vi "LabviewEnvsInstalled.vi"   [LabVIEW 2020]
uses:
  <vilib>/Wiresmith Technology/G CLI/Argument Parser/Option Class/Option Configuration.ctl
  <vilib>/Wiresmith Technology/G CLI/Argument Parser/Option Class/Argument Type.ctl
  <vilib>/Utility/error.llb/DialogType.ctl
  094f6021-4ef8-4573-82ce-a7b4949f6c5c.vi
  67a138f0-9744-4b2d-9c21-223ad79f4533.vi
  6795289f-0a04-455c-a499-a5e59a361415.vi
  <vilib>/JDP Science/JSONtext/Variant to JSON Text.vi
  <vilib>/JDP Science/JSONtext/LVClass Serializer/JSONtext LVClass Serializer.lvclass
  <vilib>/Wiresmith Technology/G CLI/CLI Class/CLI.lvclass
  <vilib>/Wiresmith Technology/G CLI/Argument Parser/Option Set Class/Option Set.lvclass
  <vilib>/Wiresmith Technology/G CLI/Argument Parser/Option Class/Option.lvclass
  <vilib>/JDP Science/JSONtext/JSONtext.lvlib
types:
  T1 = enum32{"Invalid", "Standard", "Closed", "Hidden", "Minimized", "Maximized"}
  T2 = typedef "Option Parser.lvlib/Option.lvclass/Option Configuration.ctl" = cluster{"Option Type":T3, "Option Labels":string[], "Key":string, "Description":string, "Required":bool, "Default Value":string}
  T3 = typedef "Option Parser.lvlib/Option.lvclass/Argument Type.ctl" = enum16{"flag", "value"}
  T4 = typedef "LabViewApplication--cluster.ctl" = cluster{"Bitness":enum8{"Unknown", "x86", "x64"}, "Version":string, "LabVIEW.exe":path, "VersionString":string}
  T5 = typedef "DialogType.ctl" = u16
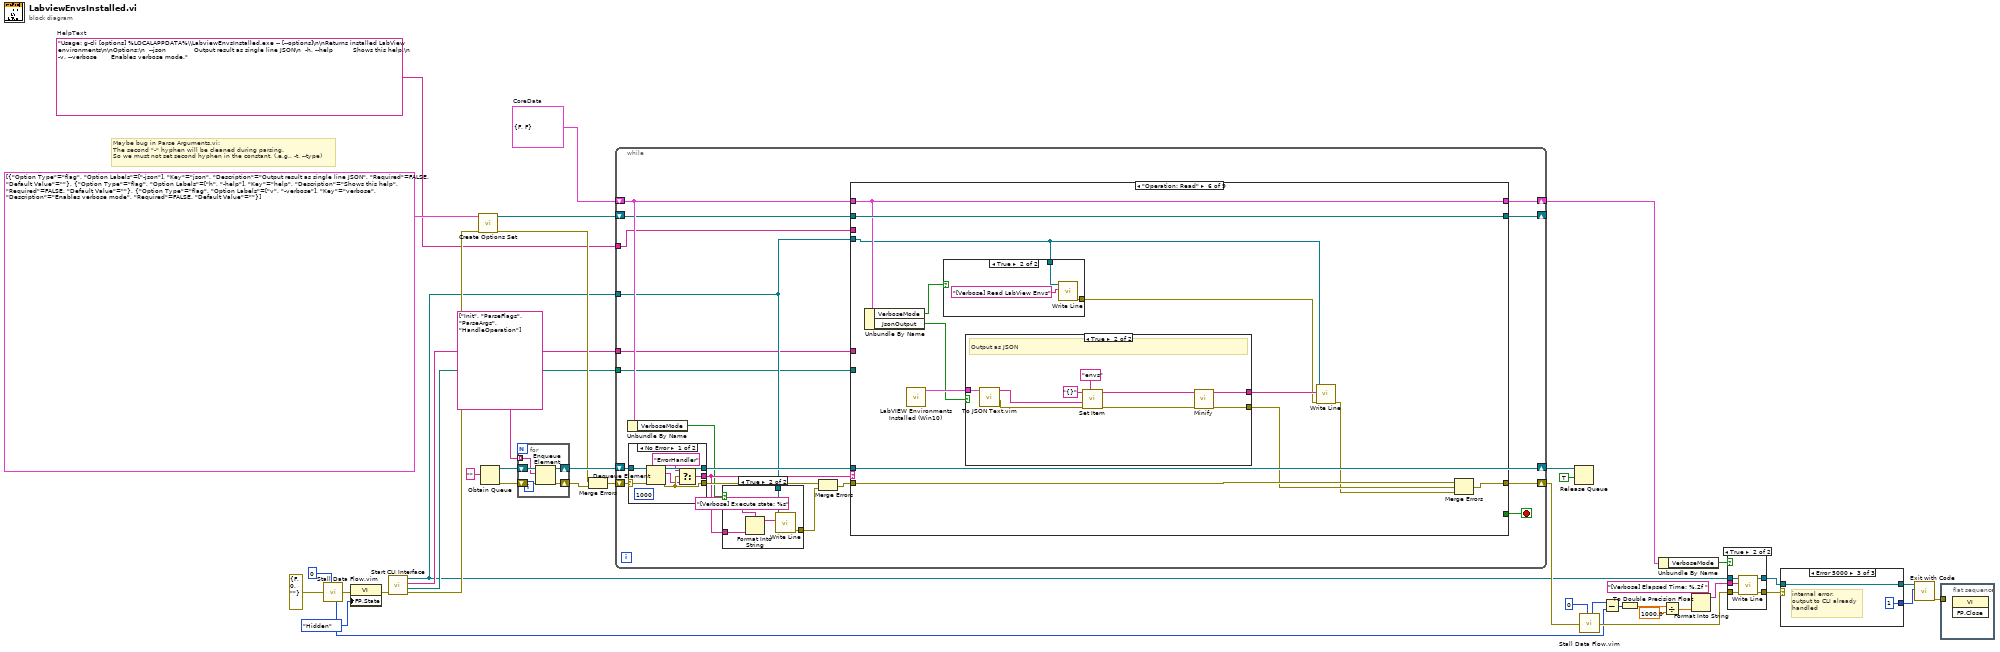
[diagram p0: block diagram]
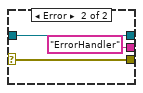
[diagram p4: hidden frame]
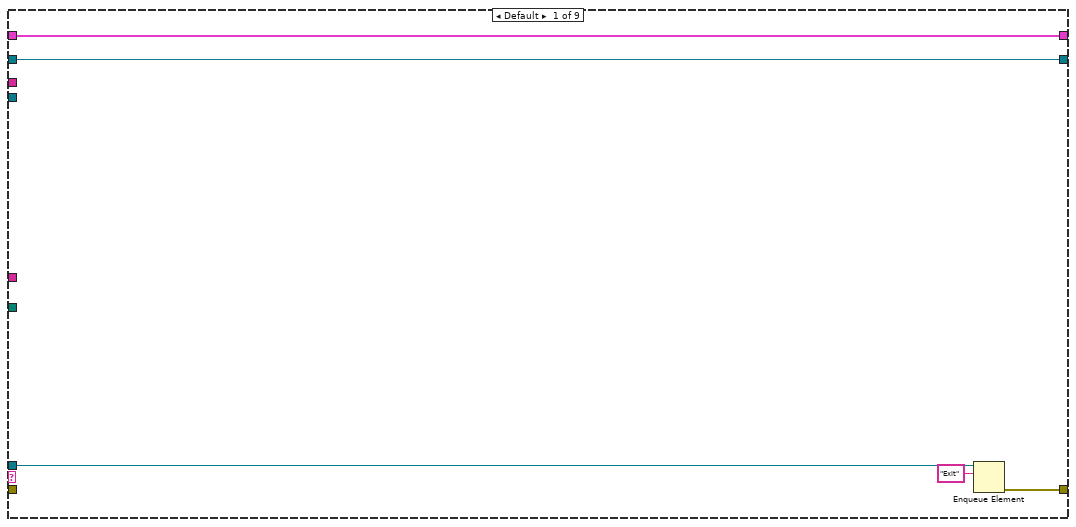
[diagram p5: hidden frame]
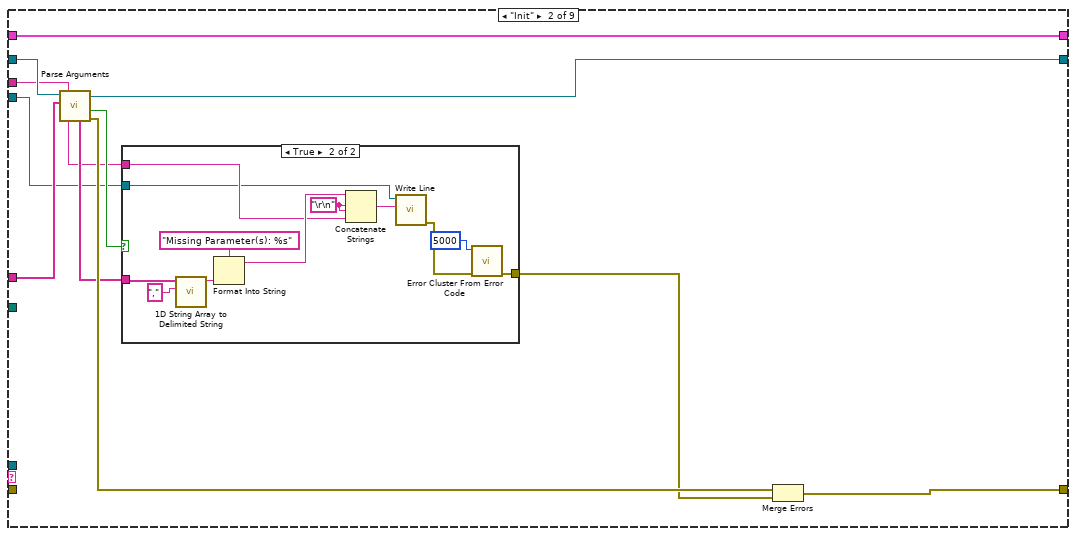
[diagram p6: hidden frame]
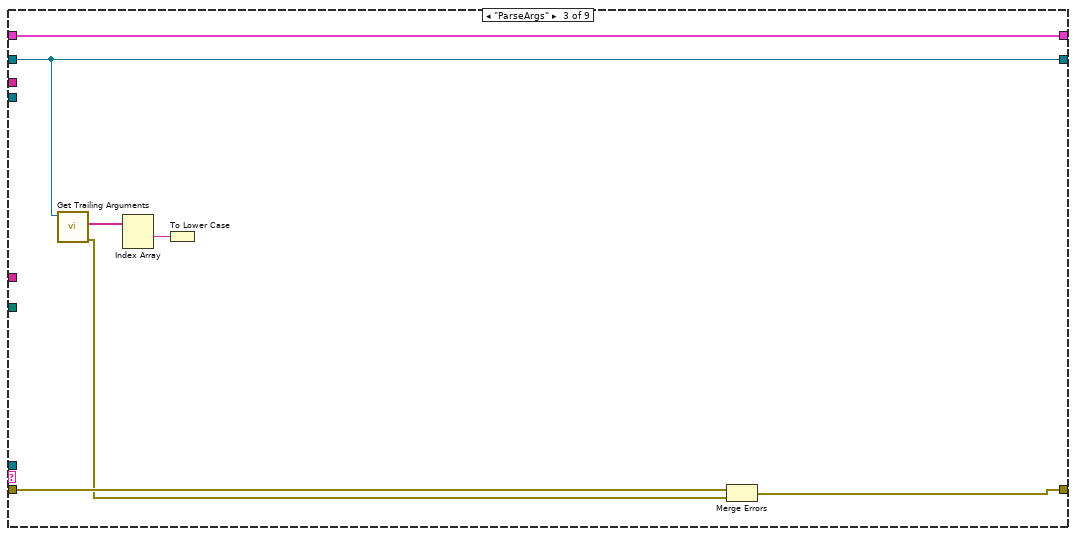
[diagram p8: hidden frame]
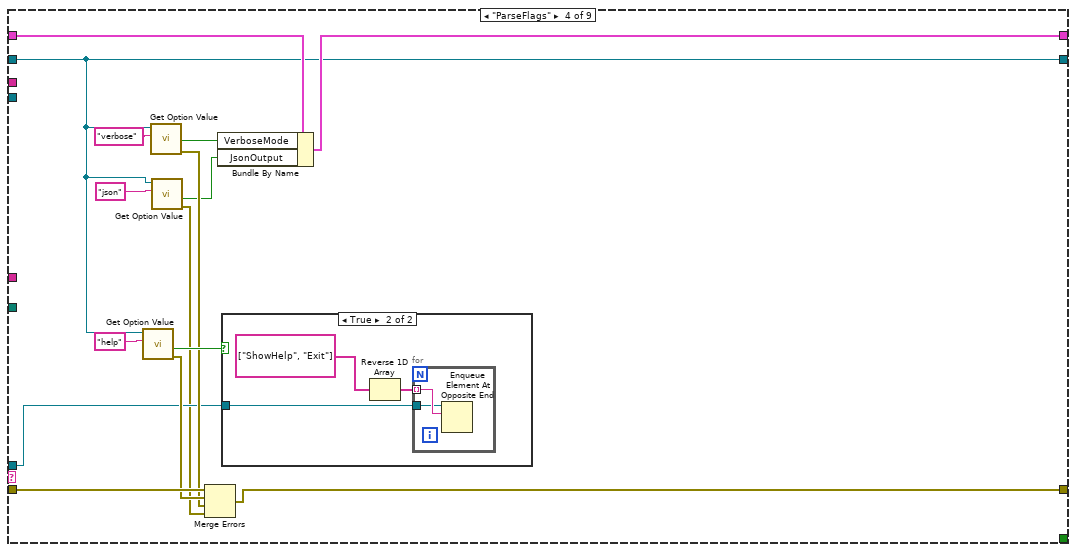
[diagram p9: hidden frame]
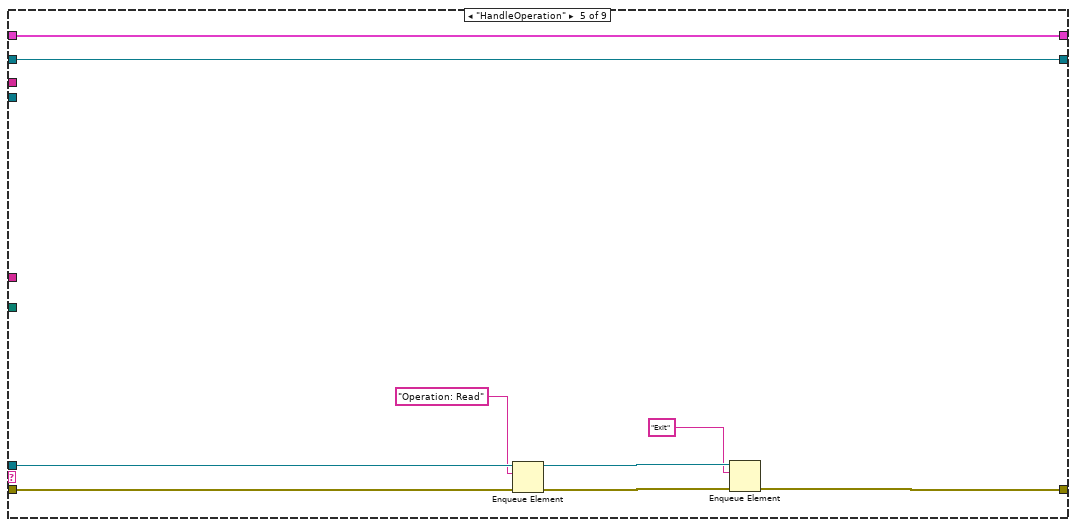
[diagram p11: hidden frame]
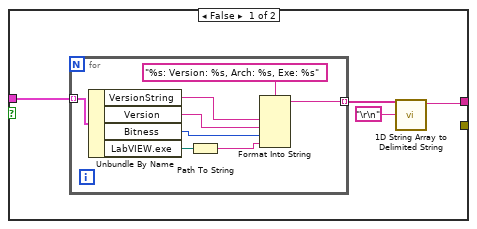
[diagram p12: hidden frame]
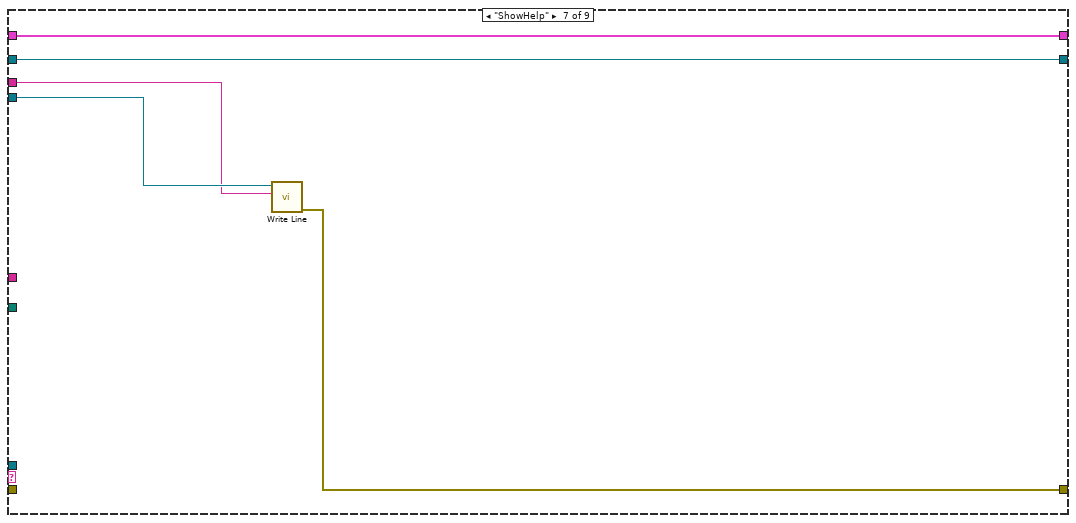
[diagram p14: hidden frame]
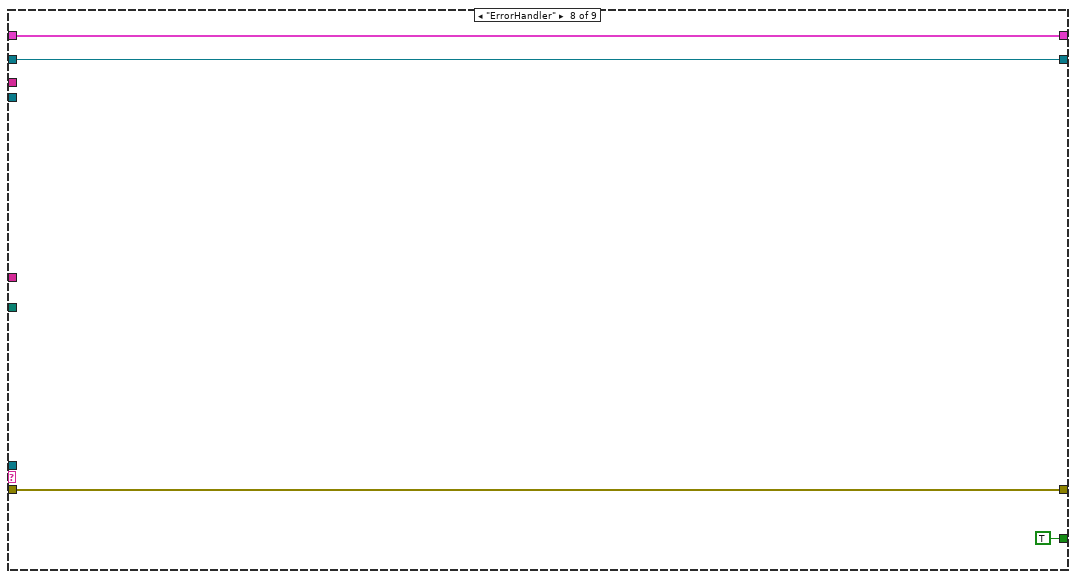
[diagram p15: hidden frame]
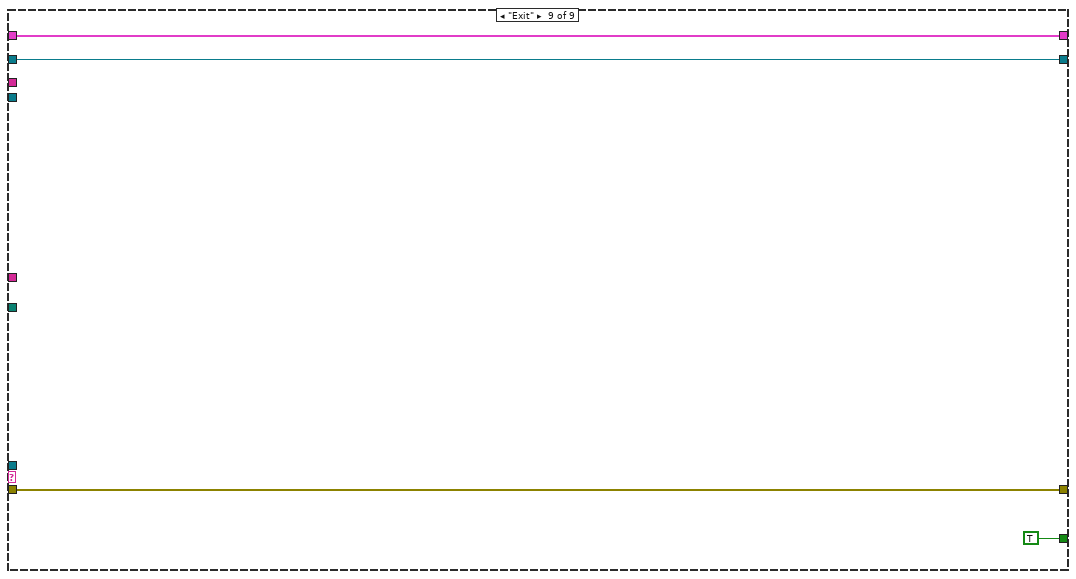
[diagram p16: hidden frame]
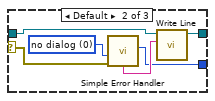
[diagram p18: hidden frame]
diagram:
  w1 = "Usage: g-cli [options] %LOCALAPPDATA%\\LabviewEnvsInstalled.exe -- [--options]\n\nReturns installed LabView environments\n\nOptions:\n  --json              Output result as single line JSON\n  -h, --help          Shows this help.\n  -v, --verbose       Enables verbose mode."  # HelpText
  w14 = cluster{"VerboseMode":bool, "JsonOutput":bool} {"VerboseMode"=FALSE, "JsonOutput"=FALSE}  # CoreData
  # "Maybe bug in Parse Arguments.vi: \nThe second \"-\" hyphen will be cleaned during parsing.\nSo we must not set second hyphen in the constant. (.e.g., -t, --type)"
  n1 = call "Stall Data Flow.vim"("value in"=errorcluster {"status"=FALSE, "code"=0, "source"=""} ("error in (no error)"), "milliseconds to wait"=u32 0) -> ("millisecond timer value"=w30:u32, "value out"=w37:errorcluster)
  n2 = property class="VI"(error in=w37, "FP.State"=T1."Hidden" ("Front Panel Window:State")) -> (error out=w36:errorcluster)  [unwired: 1 in, 1 out]
  n3 = call <vilib>:"Start CLI Interface.vi"("error in (no error)"=w36) -> ("error out"=w41:errorcluster, "Working Directory"=w7:path, "Custom Parameters"=w8:string[], "CLI out"=w5:refnum<class "CLI.lvclass">)  [unwired: 7 in]
  n4 = call <vilib>:"Create Options Set.vi"("error in (no error)"=w41, "Options"=T2[] [{"Option Type"=enum."flag", "Option Labels"=["-json"], "Key"="json", "Description"="Output result as single line JSON", "Required"=FALSE, "Default Value"=""}, {"Option Type"=enum."flag", "Option Labels"=["h", "-help"], "Key"="help", "Description"="Shows this help", "Required"=FALSE, "Default Value"=""}, {"Option Type"=enum."flag", "Option Labels"=["v", "-verbose"], "Key"="verbose", "Description"="Enables verbose mode", "Required"=FALSE, "Default Value"=""}]) -> ("error out"=w10:errorcluster, "Option Set out"=w12:refnum<class "Option Set.lvclass">)  [unwired: 8 in]
  n5 = Obtain Queue(element data type="") -> (queue out=w19:refnum<queue>, error out=w16:errorcluster)  [unwired: 4 in, 1 out]
  n6 = for {
    shift-right: [w45] -> w17
    shift-left: w19 -> [w46]
    shift-right: [w43] -> w11
    shift-left: w16 -> [w44]
    tunnel: string[] ["Init", "ParseFlags", "ParseArgs", "HandleOperation"] -> [w42] mode=indexing
    n7 = Enqueue Element(queue=w46, element=w42, error in (no error)=w44) -> (queue out=w45:refnum<queue>, error out=w43:errorcluster)  [unwired: 1 in, 1 out]
  }
  n8 = Merge Errors(w10, w11) -> (w9:errorcluster)
  n9 = while {
    shift-right: [w61] -> w4
    shift-left: w14 -> [w56]
    shift-right: [w59] -> w6
    shift-left: w9 -> [w63]
    shift-right: [w58] -> w15
    shift-left: w17 -> [w64]
    tunnel: w5 -> [w54]
    tunnel: w8 -> [w49]
    tunnel: w7 -> [w50]
    tunnel: w1 -> [w48]
    shift-right: [w47] -> _
    shift-left: w12 -> [w53]
    stop <- w60 stop-if-true
    n10 = Unbundle By Name(w56) -> ("VerboseMode"=w55:bool)
    n11 = case shown="No Error" w63 {
      selector: w63 -> [w75 w79]
      tunnel: w64 -> [w76 w78]
      tunnel: [w71 "ErrorHandler"] -> w57
      tunnel: [w73 w79] -> w62
      tunnel: [w74 w78] -> w58
      frame No Error {
        (unwired) 1000 ("timeout in ms (-1)")
        n12 = Dequeue Element(queue=w76, error in (no error)=w75) -> (queue out=w74:refnum<queue>, element=w72:string, error out=w73:errorcluster)  [unwired: 1 in, 1 out]
        n13 = Select(t="ErrorHandler", s=w73, f=w72) -> (s? t:f=w71:string)
      }
      frame Error {
      }
    }
    n14 = case shown="True" w55 {
      tunnel: w57 -> [_ w69]
      tunnel: w54 -> [_ w66]
      tunnel: [_ w65] -> w51
      frame False {
      }
      frame True {
        n15 = Format Into String(format string="[Verbose] Execute state: %s", w69) -> (resulting string=w67:string)  [unwired: 2 in, 1 out]
        n16 = call <vilib>:"Write Line.vi"("Text to Write"=w67, "CLI in"=w66) -> ("error out"=w65:errorcluster)  [unwired: 8 in, 1 out]
      }
    }
    n17 = Merge Errors(w62, w51) -> (w52:errorcluster)
    n18 = case shown="\"Operation: Read\"" w57 {
      tunnel: w52 -> [_ _ w113 w126 w141 w153 _ w187 w190]
      tunnel: [w84 w95 w114 w119 w142 w154 w184 w188 w192] -> w61
      tunnel: w56 -> [w84 w95 w114 w129 w142 w154 w184 w188 w192]
      tunnel: [_ _ _ _ _ _ _ TRUE TRUE] -> w60
      tunnel: [w82 w87 w109 w124 w136 w152 w180 w187 w190] -> w59
      tunnel: w58 -> [w83 _ _ w120 w140 _ _ _ _]
      tunnel: w54 -> [_ w88 _ _ _ w150 w182 _ _]
      tunnel: w53 -> [w80 w94 w112 w117 w143 w155 w183 w185 w189]
      tunnel: w50 -> [_ _ _ _ _ _ _ _ _]
      tunnel: w49 -> [_ w93 _ _ _ _ _ _ _]
      tunnel: w48 -> [_ w89 _ _ _ _ w181 _ _]
      tunnel: [w80 w85 w112 w117 w143 w155 w183 w185 w189] -> w47
      frame Default {
        n19 = Enqueue Element(queue=w83, element="Exit") -> (error out=w82:errorcluster)  [unwired: 2 in, 2 out]
      }
      frame "Init" {
        n20 = call <vilib>:"Parse Arguments.vi"("Arguments"=w93, "Option Set in"=w94) -> ("error out"=w92:errorcluster, "Missing Options"=w91:bool, "Option Set out"=w85:refnum<class "Option Set.lvclass">, "Missing Option Keys"=w90:string[])  [unwired: 6 in]
        n21 = case shown="True" w91 {
          tunnel: w90 -> [_ w106]
          tunnel: w89 -> [_ w101]
          tunnel: w88 -> [_ w99]
          tunnel: [_ w96] -> w86
          frame False {
          }
          frame True {
            w103 = "\r\n"
            n22 = call <vilib>:"1D String Array to Delimited String.vi"("delimiter"=",", "string array"=w106) -> ("delimited string"=w104:string)  [unwired: 9 in]
            n23 = Format Into String(format string="Missing Parameter(s): %s", w104) -> (resulting string=w102:string)  [unwired: 2 in, 1 out]
            n24 = Concatenate Strings(w102, w103, w103, w101) -> (w100:string)
            n25 = call <vilib>:"Write Line.vi"("Text to Write"=w100, "CLI in"=w99) -> ("error out"=w97:errorcluster)  [unwired: 8 in, 1 out]
            n26 = call <vilib>:"Error Cluster From Error Code.vi"("error in (no error)"=w97, "error code (0)"=5000) -> ("error out"=w96:errorcluster)  [unwired: 7 in]
          }
        }
        n27 = Merge Errors(w92, w86) -> (w87:errorcluster)
      }
      frame "ParseArgs" {
        n28 = call <vilib>:"Get Trailing Arguments.vi"("Option Set in"=w112) -> ("error out"=w108:errorcluster, "Arguments"=w111:string[])  [unwired: 8 in, 1 out]
        n29 = Index Array(array=w111) -> (element #1=w110:string)  [unwired: 2 in, 1 out]
        n30 = To Lower Case(string=w110) -> ()  [unwired: 1 out]
        n31 = Merge Errors(w113, w108) -> (w109:errorcluster)
      }
      frame "ParseFlags" {
        n32 = call <vilib>:"Get Option Value.vi"("Option Key"="help", "Option Set in"=w117) -> ("error out"=w123:errorcluster, "Set"=w127:bool)  [unwired: 6 in, 2 out]
        n33 = call <vilib>:"Get Option Value.vi"("Option Key"="verbose", "Option Set in"=w117) -> ("error out"=w122:errorcluster, "Set"=w121:bool)  [unwired: 6 in, 2 out]
        n34 = call <vilib>:"Get Option Value.vi"("Option Key"="json", "Option Set in"=w117) -> ("error out"=w116:errorcluster, "Set"=w115:bool)  [unwired: 6 in, 2 out]
        n35 = Merge Errors(w126, w123, w122, w116) -> (w124:errorcluster)
        n36 = Bundle By Name(cluster=w129, "VerboseMode"=w121, "JsonOutput"=w115) -> (w119:cluster{"VerboseMode":bool, "JsonOutput":bool})
        n37 = case shown="True" w127 {
          tunnel: w120 -> [_ w131]
          frame False {
          }
          frame True {
            n38 = Reverse 1D Array(array=string[] ["ShowHelp", "Exit"]) -> (reversed array=w130:string[])
            n39 = for {
              tunnel: w130 -> [w134] mode=indexing
              tunnel: w131 -> [w133]
              n40 = Enqueue Element At Opposite End(queue=w133, element=w134) -> ()  [unwired: 2 in, 3 out]
            }
          }
        }
      }
      frame "HandleOperation" {
        n41 = Enqueue Element(queue=w140, element="Operation: Read", error in (no error)=w141) -> (queue out=w138:refnum<queue>, error out=w139:errorcluster)  [unwired: 1 in, 1 out]
        n42 = Enqueue Element(queue=w138, element="Exit", error in (no error)=w139) -> (error out=w136:errorcluster)  [unwired: 1 in, 2 out]
      }
      frame "Operation: Read" {
        n43 = Unbundle By Name(w154) -> ("VerboseMode"=w151:bool, "JsonOutput"=w145:bool)
        n44 = call "LabVIEW Environments Installed (Win10).vi"() -> ("LabVIEW Applications Installed"=w149:T4[])  [unwired: 9 in, 2 out]
        n45 = case shown="True" w151 {
          tunnel: w150 -> [_ w179]
          tunnel: [_ w178] -> w144
          frame False {
          }
          frame True {
            n46 = call <vilib>:"Write Line.vi"("Text to Write"="[Verbose] Read LabView Envs" ("format string"), "CLI in"=w179) -> ("error out"=w178:errorcluster)  [unwired: 8 in, 1 out]
          }
        }
        n47 = case shown="True" w145 {
          tunnel: w149 -> [w159 w176]
          tunnel: [_ w175] -> w148
          tunnel: [w157 w174] -> w147
          frame False {
            n48 = for {
              tunnel: w159 -> [w167] mode=indexing
              tunnel: [w160] -> w158 mode=indexing
              n49 = Unbundle By Name(w167) -> ("VersionString"=w162:string, "Version"=w163:string, "Bitness"=w164:enum8{"Unknown", "x86", "x64"}, "LabVIEW.exe"=w166:path)
              n50 = Path To String(path=w166) -> (string=w165:string)
              n51 = Format Into String(format string="%s: Version: %s, Arch: %s, Exe: %s", w162, w163, w164, w165) -> (resulting string=w160:string)  [unwired: 2 in, 1 out]
            }
            n52 = call <vilib>:"1D String Array to Delimited String.vi"("delimiter"="\r\n", "string array"=w158) -> ("delimited string"=w157:string)  [unwired: 9 in]
          }
          frame True {
            # "Output as JSON"
            n53 = call "To JSON Text.vim"("Anything"=w176) -> ("error out"=w172:errorcluster, "<JSON>"=w173:string)  [unwired: 9 in]
            n54 = call <vilib>:"Set Item.vi"("$Path or Item Name"="envs", "error in (no error)"=w172, "JSON to Insert"=w173, "JSON"="{}") -> ("error out"=w171:errorcluster, "<JSON>"=w169:string)  [unwired: 4 in, 1 out]
            n55 = call <vilib>:"Minify.vi"("error in (no error)"=w171, "JSON"=w169) -> ("error out"=w175:errorcluster, "<JSON>"=w174:string)  [unwired: 7 in, 1 out]
          }
        }
        n56 = call <vilib>:"Write Line.vi"("error in (no error)"=w144, "Text to Write"=w147, "CLI in"=w150) -> ("error out"=w146:errorcluster)  [unwired: 7 in, 1 out]
        n57 = Merge Errors(w153, w148, w146) -> (w152:errorcluster)
      }
      frame "ShowHelp" {
        n58 = call <vilib>:"Write Line.vi"("Text to Write"=w181, "CLI in"=w182) -> ("error out"=w180:errorcluster)  [unwired: 8 in, 1 out]
      }
      frame "ErrorHandler" {
      }
      frame "Exit" {
      }
    }
  }
  n59 = Release Queue(queue=w15, force destroy? (F)=TRUE) -> ()  [unwired: 1 in, 3 out]
  n60 = call "Stall Data Flow.vim"("value in"=w6, "milliseconds to wait"=u32 0) -> ("millisecond timer value"=w31:u32, "value out"=w39:errorcluster)
  n61 = Subtract(x=w31, y=w30) -> (x-y=w29:u32)
  n62 = To Double Precision Float(number=w29) -> (double precision float=w28:dbl)
  n63 = Unbundle By Name(w4) -> ("VerboseMode"=w3:bool)
  n64 = Divide(x=w28, y=1000.0) -> (x/y=w26:dbl)
  n65 = Format Into String(format string="[Verbose] Elapsed Time: %.2f ", w26) -> (resulting string=w24:string)  [unwired: 2 in, 1 out]
  n66 = case shown="True" w3 {
    tunnel: w39 -> [w193 w199]
    tunnel: [w193 w198] -> w38
    tunnel: w5 -> [w194 w197]
    tunnel: w24 -> [_ w196]
    tunnel: [w194 w195] -> w23
    frame False {
    }
    frame True {
      n67 = call <vilib>:"Write Line.vi"("error in (no error)"=w199, "Text to Write"=w196, "CLI in"=w197) -> ("error out"=w198:errorcluster, "CLI out"=w195:refnum<class "CLI.lvclass">)  [unwired: 7 in]
    }
  }
  n68 = case shown="Error 5000" w38 {
    selector: w38 -> [_ w206 _]
    tunnel: w23 -> [w200 w205 w207]
    tunnel: [w200 w204 w207] -> w22
    tunnel: [_ w201 1 ("code out")] -> w21
    frame No Error {
    }
    frame Default {
      w203 = T5 0 items=["no dialog", "OK message", "continue or stop message", "OK message + warnings", "continue/stop + warnings"] ("type of dialog (OK msg:1)")
      n69 = call <vilib>:"Simple Error Handler.vi"("type of dialog (OK msg:1)"=w203, "error in (no error)"=w206) -> ("code out"=w201:i32, "message"=w202:string)  [unwired: 3 in, 3 out]
      n70 = call <vilib>:"Write Line.vi"("Text to Write"=w202, "CLI in"=w205) -> ("CLI out"=w204:refnum<class "CLI.lvclass">)  [unwired: 8 in, 1 out]
    }
    frame Error {
      # "internal error, \noutput to CLI already\nhandled"
    }
  }
  n71 = call <vilib>:"Exit with Code.vi"("Exit Code (0)"=w21, "CLI in"=w22) -> ("error out"=w35:errorcluster)  [unwired: 9 in]
  n72 = flat-sequence {
    tunnel: w35 -> [_]
    frame #0 {
      n73 = invoke class="VI" method="FP.Close"() -> ()  [unwired: 3 in, 3 out]
    }
  }
